vi "Raise Navigation Complete Event.vi"(4 "Event in":refnum<user-event>, 5 "Event Data":cluster{"sender":refnum<k24>, "e":refnum<k24>}, 6 "Control Ref":refnum<k24>, 7 "Event Common Data":T1) -> ()   [LabVIEW 2024, in "WebView.lvclass"]
uses:
  WebView.lvclass
  <vilib>/sklein/WebView2/Libs/Microsoft.Web.WebView2.Core.dll
  Navigation Complete Event Data--cluster.ctl
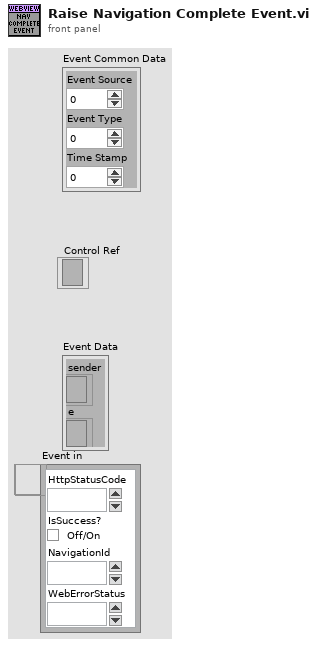
[diagram p1: front panel]
types:
  T1 = cluster{"Event Source":i32, "Event Type":u32, "Time Stamp":u32}
  T2 = typedef "WebView.lvclass/Navigation Complete Event Data--cluster.ctl" = cluster{"HttpStatusCode":i32, "IsSuccess?":bool, "NavigationId":u64, "WebErrorStatus":i32}
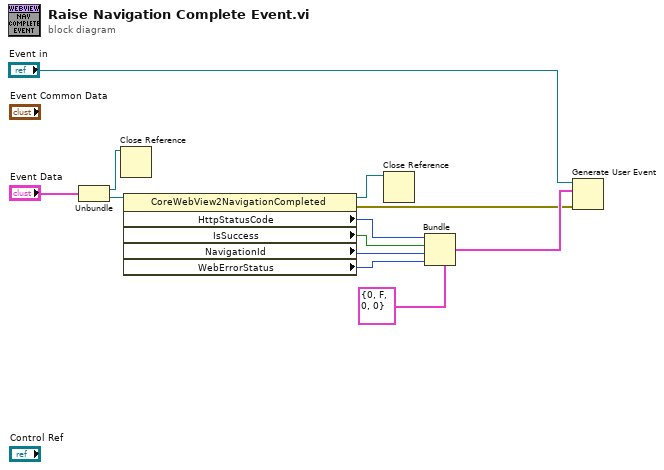
[diagram p0: block diagram]
diagram:
  n1 = Unbundle("Event Data") -> ("sender"=w3:refnum<k24>, "e"=w11:refnum<k24>)
  n2 = Close Reference(reference=w3) -> ()  [unwired: 1 in, 1 out]
  n3 = property class="CoreWebView2NavigationCompleted"(reference=w11) -> (reference out=w2:refnum<k24>, error out=w4:errorcluster, "HttpStatusCode"=w10:i32, "IsSuccess"=w9:bool, "NavigationId"=w8:u64, "WebErrorStatus"=w7:i32)  [unwired: 1 in]
  n4 = Close Reference(reference=w2) -> ()  [unwired: 1 in, 1 out]
  n5 = Bundle(cluster=T2 {"HttpStatusCode"=0, "IsSuccess?"=FALSE, "NavigationId"=0, "WebErrorStatus"=0} ("output cluster"), "HttpStatusCode"=w10, "IsSuccess?"=w9, "NavigationId"=w8, "WebErrorStatus"=w7) -> (w5:T2)
  n6 = Generate User Event(user event="Event in", event data cluster=w5, error in=w4) -> ()  [unwired: 1 in, 2 out]
